vi "Reset Test Status.vi"(8 "error in (no error)":errorcluster, 11 "Model in":refnum<class "Model.lvclass">) -> (0 "error out":errorcluster, 3 "Model out":refnum<class "Model.lvclass">)   [LabVIEW 2016]
uses:
  Typedefs/TestStatus.ctl
  Typedefs/HPMT_Typedefs.lvlib
  Typedefs/AllTestStatus.ctl
  Model.lvclass
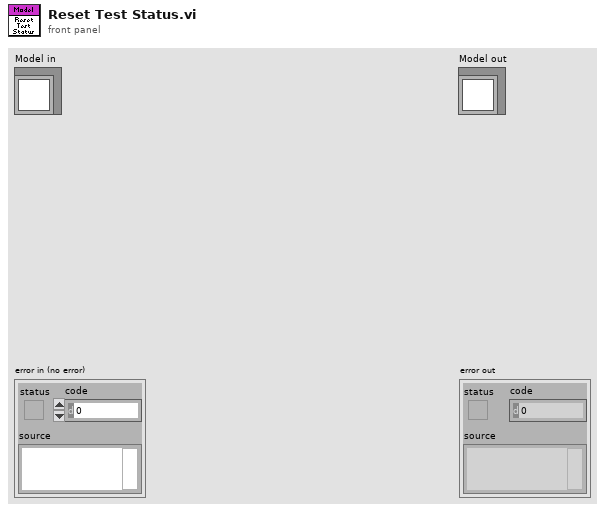
[diagram p1: front panel]
types:
  T1 = typedef "HPMT_Typedefs.lvlib/AllTestStatus.ctl" = cluster{"Test One":T2}
  T2 = typedef "HPMT_Typedefs.lvlib/TestStatus.ctl" = enum16{"Not Run", "Running", "Passed", "Failed"}
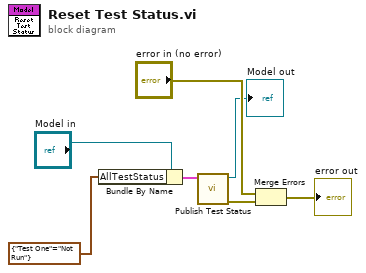
[diagram p0: block diagram]
diagram:
  n1 = Bundle By Name(cluster="Model in", "AllTestStatus"=T1 {"Test One"=enum."Not Run"}) -> (w3:cluster{})
  n2 = call "Publish Test Status.vi"("Model in"=w3) -> ("error out"=w1:errorcluster, "Model out"=→"Model out":refnum<class "Model.lvclass">)  [unwired: 9 in]
  n3 = Merge Errors("error in (no error)", w1) -> (→"error out":errorcluster)
